vi "Motic Set Mirror.vi"(8 "error in (no error)":errorcluster, 10 "b":bool, 11 "camera":i32) -> (0 "error out":errorcluster, 3 "camera out":i32)   [LabVIEW 2012, in "MoticApi.lvlib"]
doc: "MOTICAPI bool Motic_SetMirror(MUCam_Handle camera, bool b);"
uses:
  MoticApi.lvlib
  MoticApi.dll
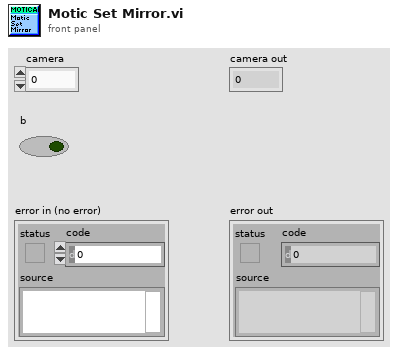
[diagram p1: front panel]
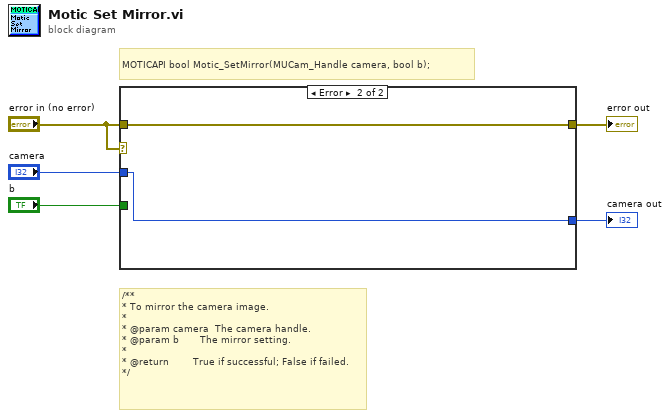
[diagram p0: block diagram]
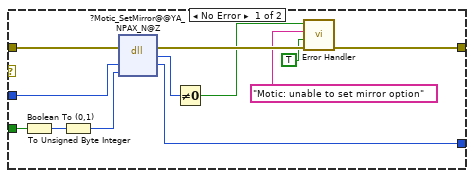
[diagram p2: hidden frame]
diagram:
  # "/**\n* To mirror the camera image.\n*\n* @param camera  The camera handle.\n* @param b       The mirror setting.\n*\n* @return        True if successful; False if failed.\n*/"
  # "MOTICAPI bool Motic_SetMirror(MUCam_Handle camera, bool b);"
  n1 = case shown="Error" "error in (no error)" {
    tunnel: "camera" -> [w17 w18]
    tunnel: [w16 w18] -> w4
    tunnel: "b" -> [w15 _]
    tunnel: "error in (no error)" -> [w14 w19]
    tunnel: [w12 w19] -> w2
    frame No Error {
      n2 = Boolean To (0,1)(Boolean=w15) -> (0, 1=w7:i16)
      n3 = To Unsigned Byte Integer(number=w7) -> (unsigned 8bit integer=w6:u8)
      n4 = dll-call lib="C:/Users/TTS-Digital/Desktop/MoticApi/MoticApi_git/MoticApi/MoticApi.*" fn="?Motic_SetMirror@@YA_NPAX_N@Z"(error in=w14, "camera"=w17, "b"=w6) -> (error out=w13:errorcluster, w11:u8, "camera"=w16:i32)  [unwired: 3 in, 1 out]
      n5 = Not Equal To 0?(x=w11) -> (x != 0?=w10:bool)
      n6 = call "Error Handler.vi"("error in (no error)"=w13, "Is warning?"=TRUE, "Error message"="Motic: unable to set mirror option", "Function return"=w10) -> ("error out"=w12:errorcluster)  [unwired: 7 in]
    }
    frame Error {
    }
  }
  "camera out" <- w4
  "error out" <- w2
